vi "GVSDataView Splitter MDown Process.vi"(6 "DataView Index":i32, 8 "Selected Spliter Ref":refnum<vi>, 9 "Bar_shadow ref":refnum<vi>, 10 "Mouse Pos":T2, 11 "SpliterMove Info":T1) -> (3 "SpliterMove Out":T1)   [LabVIEW 2013]
uses:
  GVSNew View Global.vi
panel:
  in  "sp_mdown_hei":i32
  in  "sp_mdown_wid":i32
  in  "sp_mdown_ypos":i32
  in  "sp_mdown_xpos":i32
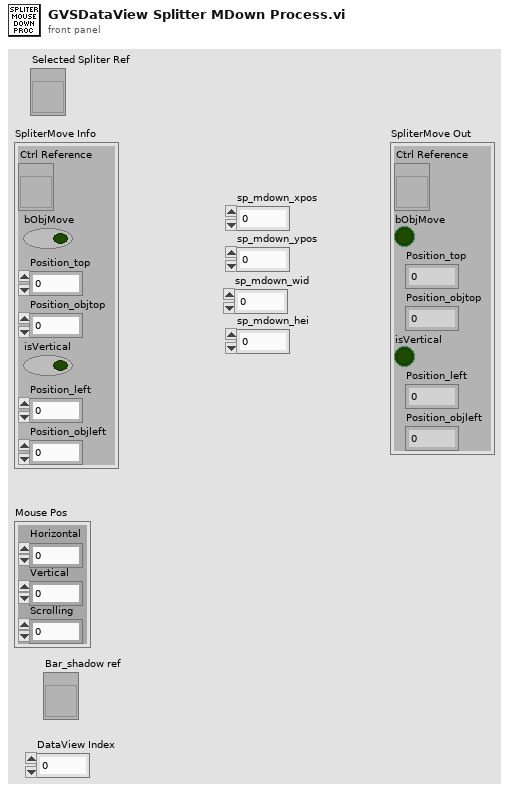
[diagram p1: front panel]
types:
  T1 = cluster{"Ctrl Reference":refnum<vi>, "bObjMove":bool, "Position_top":i32, "Position_objtop":i32, "isVertical":bool, "Position_left":i32, "Position_objleft":i32}
  T2 = cluster{"Horizontal":i32, "Vertical":i32, "Scrolling":i32}
  T3 = typedef "Graph Main Info Cluster.ctl" = cluster{"Selected_BarIdx":i32, "Selected_PanelIdx":i32, "Graph Main VIRef":refnum<vi>, "ToolBarClick":bool, "Spliter Ref Array":refnum<vi>[], "Panel Ref Array":refnum<vi>[], "Spliter_matrix":i32[][], "Panel_matrix":i32[][], "child_spliterIdx_matrix":i32[][], "split_pos_matrix":i32[][], "Title State":bool, "sQueueName":string, "Frame nID":i32, "Graph VIRef Array":cluster{"Graph VIRef":refnum<vi>, "Panel Idx":i32, "Frame VIRef":refnum<vi>, "Icon Ring":i32, "Graph Type":string}[], "View Type":string}
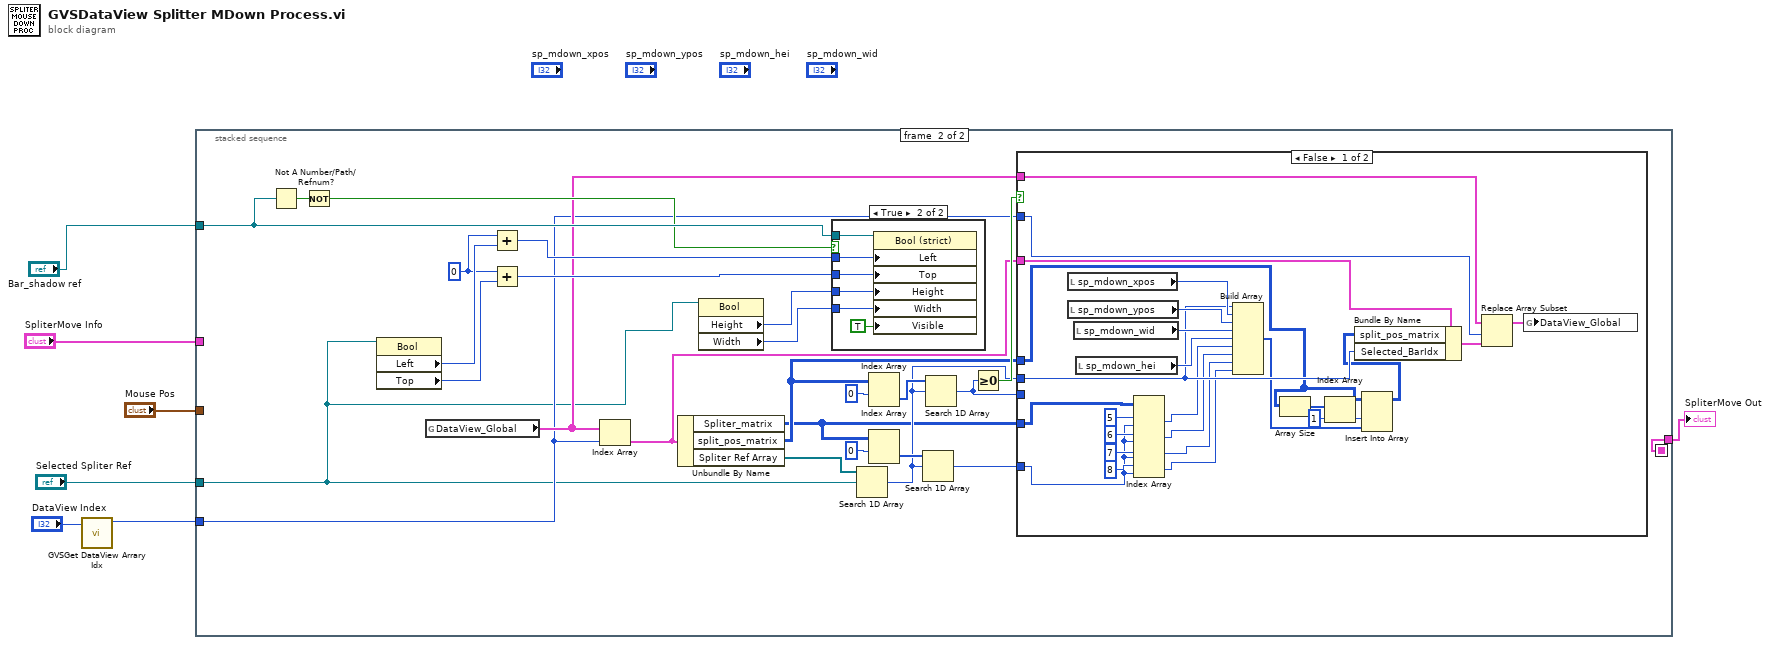
[diagram p0: block diagram]
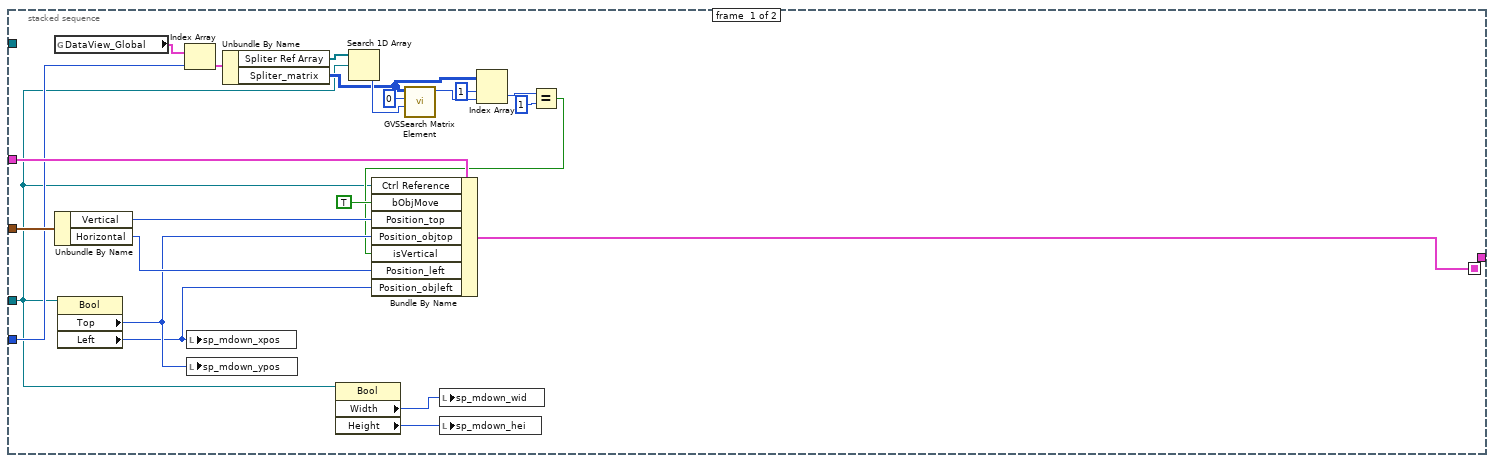
[diagram p2: hidden frame]
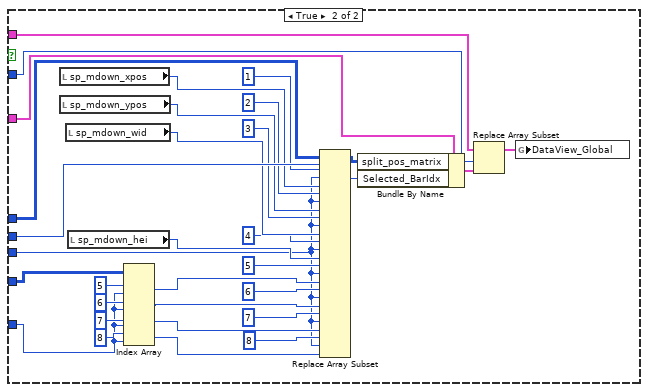
[diagram p4: hidden frame]
diagram:
  n1 = call "GVSGet DataView Arrary Idx.vi"("DataView Idx In"="DataView Index") -> ("DataView Arrary Idx out"=w2:i32)  [unwired: 10 in]
  n2 = stacked-sequence {
    seq-local: [w21 _] -> [_ w35]
    tunnel: "SpliterMove Info" -> [w28 _]
    tunnel: "Selected Spliter Ref" -> [w8 w31]
    tunnel: "Mouse Pos" -> [w22 _]
    tunnel: "Bar_shadow ref" -> [_ w39]
    tunnel: [_ w35] -> w4
    tunnel: w2 -> [w19 w32]
    frame #0 {
      n3 = global read "GVSNew View Global.vi" "DataView_Global"() -> (w20:T3[])
      n4 = Unbundle By Name(w22) -> ("Vertical"=w30:i32, "Horizontal"=w27:i32)
      n5 = property class="Bool"(reference=w8) -> ("Top"=w26:i32, "Left"=w25:i32)  [unwired: 1 in, 2 out]
      n6 = Index Array(array=w20, index=w19) -> (element=w18:T3)
      n7 = local write "sp_mdown_xpos"(w25) -> ()
      n8 = local write "sp_mdown_ypos"(w26) -> ()
      n9 = Unbundle By Name(w18) -> ("Spliter Ref Array"=w17:refnum<vi>[], "Spliter_matrix"=w14:i32[][])
      n10 = property class="Bool"(reference=w8) -> ("Width"=w23:u32, "Height"=w24:u32)  [unwired: 1 in, 2 out]
      n11 = Search 1D Array(1D array=w17, element=w8) -> (index of element=w15:i32)  [unwired: 1 in]
      n12 = call "GVSSearch Matrix Element.vi"("element"=w15, "index (row)"=0, "matrix in"=w14) -> ("index of element"=w13:i32)  [unwired: 8 in]
      n13 = local write "sp_mdown_wid"(w23) -> ()
      n14 = local write "sp_mdown_hei"(w24) -> ()
      n15 = Index Array(array=w14, index (row)=1 ("disabled index (row)"), index (col)=w13) -> (element=w11:i32)
      n16 = Equal?(x=w11, y=1) -> (x = y?=w9:bool)
      n17 = Bundle By Name(cluster=w28, "Ctrl Reference"=w8, "bObjMove"=TRUE ("객체이동"), "Position_top"=w30, "Position_objtop"=w26, "isVertical"=w9, "Position_left"=w27, "Position_objleft"=w25) -> (w21:T1)
    }
    frame #1 {
      w43 = 0 ("x")
      n18 = Not A Number/Path/Refnum?(number/path/refnum=w39) -> (NaN/Path/Refnum?=w38:bool)
      n19 = Not(x=w38) -> (.not. x?=w37:bool)
      n20 = property class="Bool"(reference=w31) -> ("Left"=w47:i32, "Top"=w45:i32)  [unwired: 1 in, 2 out]
      n21 = global read "GVSNew View Global.vi" "DataView_Global"() -> (w36:T3[])
      n22 = Add(x=w43, y=w47) -> (x+y=w46:i32)
      n23 = Add(x=w43, y=w45) -> (x+y=w44:i32)
      n24 = Index Array(array=w36, index=w32) -> (element=w42:T3)
      n25 = Unbundle By Name(w42) -> ("Spliter_matrix"=w33:i32[][], "split_pos_matrix"=w34:i32[][], "Spliter Ref Array"=w40:refnum<vi>[])
      n26 = property class="Bool"(reference=w31) -> ("Height"=w49:u32, "Width"=w48:u32)  [unwired: 1 in, 2 out]
      n27 = case shown="True" w37 {
        tunnel: w49 -> [_ w62]
        tunnel: w48 -> [_ w61]
        tunnel: w46 -> [_ w59]
        tunnel: w44 -> [_ w58]
        tunnel: w39 -> [_ w57]
        frame False {
        }
        frame True {
          n28 = property class="Bool (strict)"(reference=w57, "Left"=w59, "Top"=w58, "Height"=w62, "Width"=w61, "Visible"=TRUE) -> ()  [unwired: 1 in, 2 out]
        }
      }
      n29 = Search 1D Array(1D array=w40, element=w31) -> (index of element=w41:i32)  [unwired: 1 in]
      n30 = Index Array(array=w34, index (row)=0) -> (element=w54:i32[])  [unwired: 1 in]
      n31 = Index Array(array=w33, index (row)=0) -> (element=w51:i32[])  [unwired: 1 in]
      n32 = Search 1D Array(1D array=w51, element=w41) -> (index of element=w50:i32)  [unwired: 1 in]
      n33 = Search 1D Array(1D array=w54, element=w41) -> (index of element=w55:i32)  [unwired: 1 in]
      n34 = Greater Or Equal To 0?(x=w55) -> (x >= 0?=w56:bool)
      n35 = case shown="False" w56 {
        tunnel: w55 -> [_ w91]
        tunnel: w41 -> [w80 w115]
        tunnel: w50 -> [w73 w108]
        tunnel: w34 -> [w65 w107]
        tunnel: w33 -> [w74 w109]
        tunnel: w32 -> [w83 w117]
        tunnel: w42 -> [w82 w116]
        tunnel: w36 -> [w79 w114]
        frame False {
          n36 = local read "sp_mdown_xpos"() -> (w85:i32)
          n37 = local read "sp_mdown_ypos"() -> (w86:i32)
          n38 = local read "sp_mdown_wid"() -> (w87:i32)
          n39 = local read "sp_mdown_hei"() -> (w88:i32)
          n40 = Index Array(array=w74, index (row) #1=5 ("index (row)"), index (col) #1=w73, index (row) #2=6 ("index (row)"), index (col) #2=w73, index (row) #3=7 ("index (row)"), index (col) #3=w73, index (row) #4=8 ("index (row)"), index (col) #4=w73) -> (element #1=w72:i32, element #2=w71:i32, element #3=w70:i32, element #4=w69:i32)
          n41 = Build Array(w80, w85, w86, w87, w88, w72, w71, w70, w69) -> (w64:i32[])
          n42 = Array Size(array=w65) -> (size(s)=w68:i32[])
          n43 = Index Array(array=w68, index=1) -> (element=w66:i32)
          n44 = Insert Into Array(array=w65, index (col)=w66, new element=w64) -> (w63:i32[][])  [unwired: 1 in]
          n45 = Bundle By Name(cluster=w82, "split_pos_matrix"=w63, "Selected_BarIdx"=w80) -> (w81:T3)
          n46 = Replace Array Subset(array=w79, new element=w81, index=w83) -> (w84:T3[])
          n47 = global write "GVSNew View Global.vi" "DataView_Global"(w84) -> ()
        }
        frame True {
          n48 = local read "sp_mdown_xpos"() -> (w105:i32)
          n49 = local read "sp_mdown_ypos"() -> (w103:i32)
          n50 = local read "sp_mdown_wid"() -> (w101:i32)
          n51 = local read "sp_mdown_hei"() -> (w99:i32)
          n52 = Index Array(array=w109, index (row) #1=5 ("index (row)"), index (col) #1=w108, index (row) #2=6 ("index (row)"), index (col) #2=w108, index (row) #3=7 ("index (row)"), index (col) #3=w108, index (row) #4=8 ("index (row)"), index (col) #4=w108) -> (element #1=w97:i32, element #2=w95:i32, element #3=w93:i32, element #4=w90:i32)
          n53 = Replace Array Subset(array=w107, new element #1=w105, index (row) #1=1 ("disabled index (row)"), index (col) #1=w91, new element #2=w103, index (row) #2=2 ("disabled index (row)"), index (col) #2=w91, new element #3=w101, index (row) #3=3 ("disabled index (row)"), index (col) #3=w91, new element #4=w99, index (row) #4=4 ("disabled index (row)"), index (col) #4=w91, new element #5=w97, index (row) #5=5 ("disabled index (row)"), index (col) #5=w91, new element #6=w95, index (row) #6=6 ("disabled index (row)"), index (col) #6=w91, new element #7=w93, index (row) #7=7 ("disabled index (row)"), index (col) #7=w91, new element #8=w90, index (row) #8=8 ("disabled index (row)"), index (col) #8=w91) -> (w89:i32[][])
          n54 = Bundle By Name(cluster=w116, "split_pos_matrix"=w89, "Selected_BarIdx"=w115) -> (w118:T3)
          n55 = Replace Array Subset(array=w114, new element=w118, index=w117) -> (w119:T3[])
          n56 = global write "GVSNew View Global.vi" "DataView_Global"(w119) -> ()
        }
      }
    }
  }
  "SpliterMove Out" <- w4
